vi "LLXPC 71-146 TCP BE Stat AMP2.vi"() -> ()   [LabVIEW 2013]
panel:
  out "output cluster":T1={"Result"=6.15, "Result"=6.15, "Result"=22.7, "Result"=23.5}
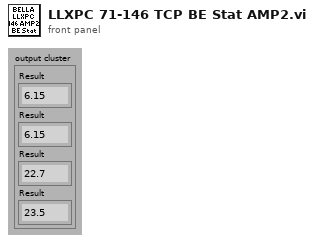
[diagram p1: front panel]
types:
  T1 = cluster{"Result":dbl, "Result":dbl, "Result":dbl, "Result":dbl}
diagram:
